vi "initialise.vi"(8 "error in (no error)":errorcluster, 11 "ExperimentControllerDL090130Interval in":refnum<class "ExperimentControllerDL090130Interval.lvclass">) -> (0 "error out":errorcluster, 3 "ExperimentControllerDL090130Interval out":refnum<class "ExperimentControllerDL090130Interval.lvclass">)   [LabVIEW 2010, in "ExperimentControllerDL090130Interval.lvclass"]
doc: "The dynamic dispatch-version of this VI initalises the plug-in object by allocating and initalising any dynamic resources need."
uses:
  ExperimentControllerDL090130Interval.lvclass
  GenericExperimentController/GenericExperimentController/GenericExperimentController.lvclass
  ExperimentControllerDL090130Interval.lvclass/ExperimentControllerDL090130Interval.ctl
  Sweep/GenericSweep/GenericSweep/GenericSweep.lvclass
  common/classes/ErrorController/ErrorController/class_data.vi
  common/classes/ErrorController/ErrorController/ErrorController.lvclass
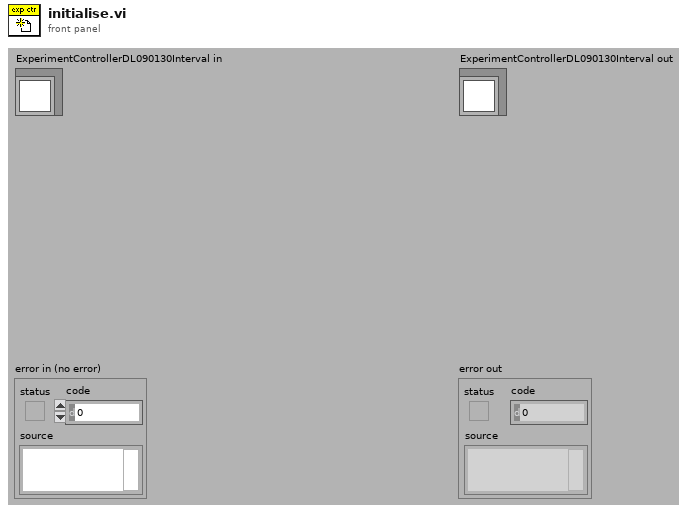
[diagram p1: front panel]
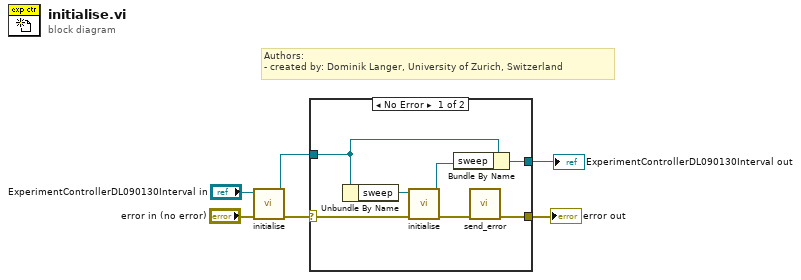
[diagram p0: block diagram]
diagram:
  # "Authors: \n- created by: Dominik Langer, University of Zurich, Switzerland"
  n1 = call-parent "initialise.vi"("error in (no error)"="error in (no error)", "GenericPlugin in"="ExperimentControllerDL090130Interval in") -> ("error out"=w4:errorcluster, "GenericPlugin out"=w3:refnum<class "ExperimentControllerDL090130Interval.lvclass">)  [unwired: 8 in]
  n2 = case shown="No Error" w4 {
    selector: w4 -> [w13 w14]
    tunnel: w3 -> [w10 w15]
    tunnel: [w7 w14] -> w2
    tunnel: [w9 w15] -> w1
    frame No Error {
      n3 = Unbundle By Name(w10) -> ("sweep"=w12:refnum<class "GenericSweep.lvclass">)
      n4 = call-dynamic "initialise.vi"("error in (no error)"=w13, "GenericPlugin in"=w12) -> ("error out"=w8:errorcluster, "GenericPlugin out"=w11:refnum<class "GenericSweep.lvclass">)  [unwired: 8 in]
      n5 = Bundle By Name(cluster=w10, "sweep"=w11) -> (w9:refnum<class "ExperimentControllerDL090130Interval.lvclass">)
      n6 = call "send_error.vi"("error in (no error)"=w8) -> ("error out"=w7:errorcluster)  [unwired: 10 in]
    }
    frame Error {
    }
  }
  "error out" <- w2
  "ExperimentControllerDL090130Interval out" <- w1
